vi "Read Measurement Data.vi"(8 "error in (no error)":errorcluster, 10 "Reading Option (0: Latest)":i32(ring) items=["Latest", "New"], 11 "VISA resource name":refnum<visa-resource-name>) -> (0 "error out":errorcluster, 2 "Measurement":T1 {"Measurement" format="%.6e"}, 3 "VISA resource name out":refnum<visa-resource-name>)   [LabVIEW 2016, in "Keithley 6517.lvlib"]
doc: "Reads the latest or a new reading from the instrument."
uses:
  <instrlib>/Keithley 6517/Keithley 6517.lvlib
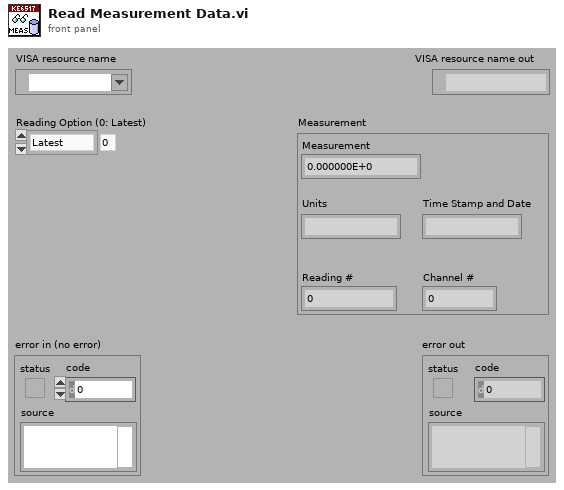
[diagram p1: front panel]
types:
  T1 = cluster{"Measurement":dbl, "Units":string, "Time Stamp and Date":string, "Reading #":dbl, "Channel #":dbl}
  T2 = typedef "Keithley 6517.lvlib/Extended User Data.ctl" = cluster{"Instrument Model":i32}
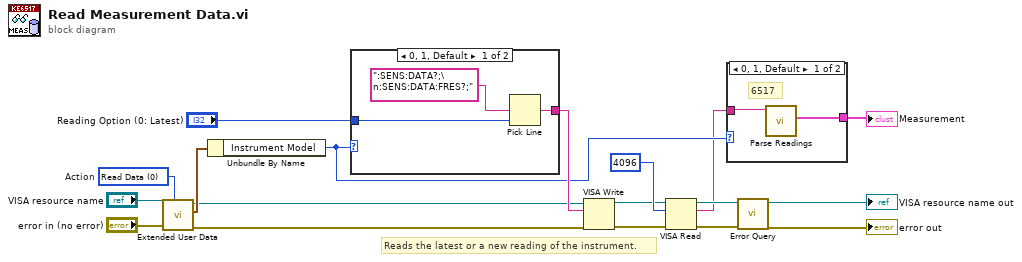
[diagram p0: block diagram]
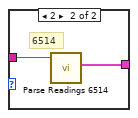
[diagram p2: hidden frame]
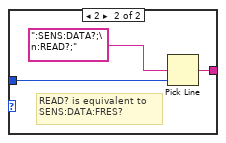
[diagram p3: hidden frame]
diagram:
  w7 = u16 0 items=["Read Data", "Write Data", "Clear Data", "Clear ALL Data"]  # Action
  # "Reads the latest or a new reading of the instrument."
  n1 = call <instrlib>:"Extended User Data.vi"("Action (0: Read Data)"=w7, "error in (no error)"="error in (no error)", "VISA resource name"="VISA resource name") -> ("error out"=w6:errorcluster, "User Data Out"=w8:T2, "VISA resource name out"=w4:refnum<visa-resource-name>)  [unwired: 6 in]
  n2 = Unbundle By Name(w8) -> ("Instrument Model"=w3:i32)
  n3 = case shown="0, 1, Default" w3 {
    tunnel: "Reading Option (0: Latest)" -> [w21 w24]
    tunnel: [w19 w22] -> w5
    frame 0, 1, Default {
      n4 = Pick Line(multi-line string=":SENS:DATA?;\n:SENS:DATA:FRES?;", line index=w21) -> (output string=w19:string)  [unwired: 1 in]
    }
    frame 2 {
      # "READ? is equivalent to\nSENS:DATA:FRES?"
      n5 = Pick Line(multi-line string=":SENS:DATA?;\n:READ?;", line index=w24) -> (output string=w22:string)  [unwired: 1 in]
    }
  }
  n6 = VISA Write(VISA resource name=w4, write buffer=w5, error in (no error)=w6) -> (VISA resource name out=w17:refnum<visa-resource-name>, error out=w16:errorcluster)  [unwired: 1 out]
  n7 = VISA Read(VISA resource name=w17, byte count=u32 4096, error in (no error)=w16) -> (VISA resource name out=w15:refnum<visa-resource-name>, read buffer=w2:string, error out=w14:errorcluster)  [unwired: 1 out]
  n8 = case shown="0, 1, Default" w3 {
    tunnel: [w26 w28] -> w1
    tunnel: w2 -> [w25 w27]
    frame 0, 1, Default {
      # "6517"
      n9 = call <instrlib>:"Parse Readings.vi"("Readings"=w25) -> ("Measurement"=w26:T1)  [unwired: 9 in, 1 out]
    }
    frame 2 {
      # "6514"
      n10 = call <instrlib>:"Parse Readings 6514.vi"("Readings"=w27) -> ("Measurement"=w28:T1)  [unwired: 9 in, 1 out]
    }
  }
  "Measurement" <- w1
  n11 = call <instrlib>:"Error Query.vi"("error in (no error)"=w14, "VISA resource name"=w15) -> ("error out"=→"error out":errorcluster, "VISA resource name out"=→"VISA resource name out":refnum<visa-resource-name>)  [unwired: 6 in, 2 out]
